vi "Verify Combinations.vi"(4 "Execution time (s)":dbl=-1.0, 5 "Assert Only? (F)":bool, 6 "error code (1)":i32=1, 7 "Options":refnum<class "Options.lvclass">, 8 "error in":errorcluster, 9 "ctl label -> value var[]":map{string, variant[]}(c390), 10 "VI Refnum":refnum<vi>, 11 "Label":string) -> (0 "error out":errorcluster, 2 "Properties":refnum<class "Properties.Assert.lvclass">)   [LabVIEW 2020, in "Caraya.Extension.lvlib"]
doc: "This is similar to the verify parameterized (in fact it calls it behind the scenes). Instead of specifying each set of parameters, you specify a single map which maps each control label to an array of variant values (there is a utility vi, \"array to array of variants.vim) to assist with this. From this, the verify function calculates each set of parameters from all the possible combinations and verifyies each combination."
uses:
  Caraya.Extension.lvlib
  <vilib>/addons/_JKI Toolkits/Caraya/classes/Properties.Assert/Properties.Assert.lvclass
  Approval Tests/Options/Options.lvclass/Options.ctl
  Approval Tests/Naming Data/Naming Data.lvclass/Naming Data.ctl
  <vilib>/addons/_JKI Toolkits/Caraya/classes/Assert/Assert.lvclass
  <vilib>/addons/_JKI Toolkits/Caraya/classes/Assert/Assert True.vi
  Approval Tests/Options/Options.lvclass
  Approval Tests/Approval Tests.lvlib
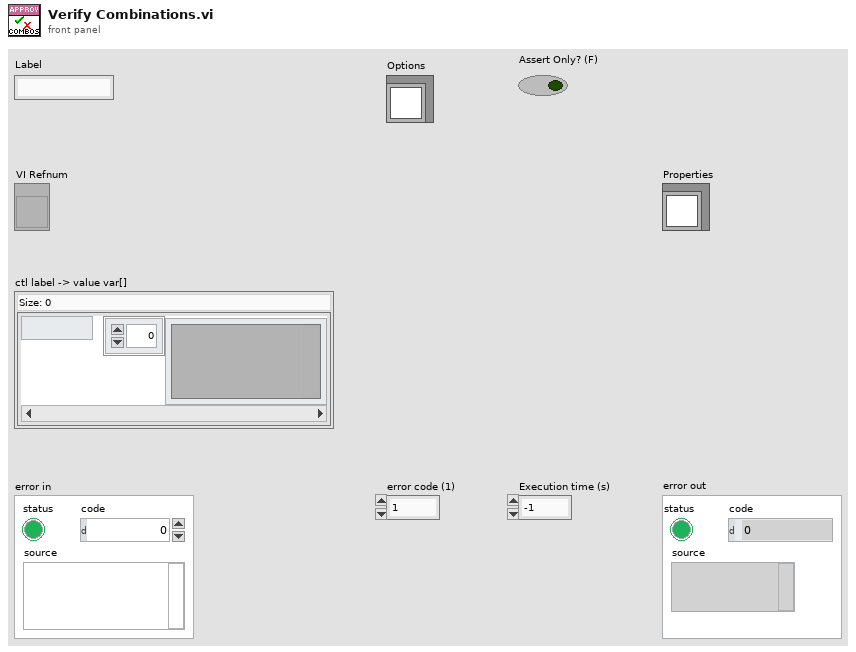
[diagram p1: front panel]
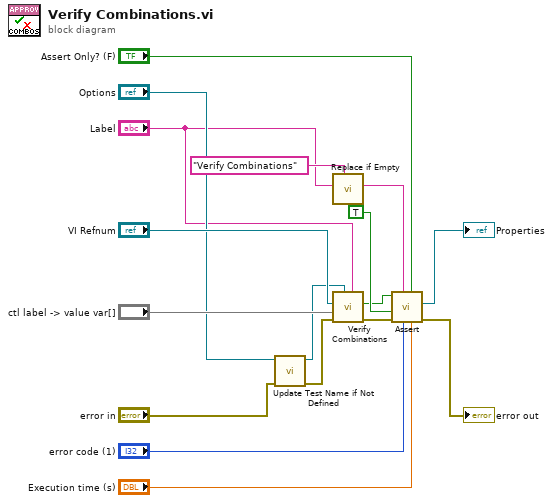
[diagram p0: block diagram]
diagram:
  n1 = call "Update Test Name if Not Defined.vi"("error in"="error in", "Options in"="Options") -> ("error out"=w14:errorcluster, "Options out"=w4:refnum<class "Options.lvclass">)  [unwired: 8 in]
  n2 = call "Replace if Empty.vi"("if empty"="Verify Combinations" ("Label"), "Text in"="Label") -> ("Text out"=w2:string)  [unwired: 9 in]
  n3 = call "Verify Combinations.vi"("Label"="Label", "Approval Tests.lvlib:Options.lvclass"=w4, "error in"=w14, "ctl label -> value var[]"="ctl label -> value var[]", "VI Refnum"="VI Refnum") -> ("error out"=w15:errorcluster, "Passed?"=w10:bool)  [unwired: 4 in, 1 out]
  n4 = call-poly <vilib>:"Assert.vi"("Execution time (s)"="Execution time (s)", "Assert Only? (F)"="Assert Only? (F)", "error code (1)"="error code (1)", "Label"=w2, "error in (no error)"=w15, "Register with caller test (F)"=TRUE, "True?"=w10) -> ("error out"=→"error out":errorcluster, "Properties"=→"Properties":refnum<class "Properties.Assert.lvclass">)  [unwired: 3 in]
